vi "Get_WebService_Data.vi"(8 "error in (no error)":errorcluster, 11 "Class in":refnum<class "AB_WebService.lvclass">) -> (0 "error out":errorcluster, 2 "data":T1, 3 "class out":refnum<class "AB_WebService.lvclass">)   [LabVIEW 2020, in "AB_WebService.lvclass"]
uses:
  <vilib>/AppBuilder/AB_Classes/WebService/AB_WebService.lvclass
  <vilib>/AppBuilder/AB_Classes/WebService/AB_WebService.ctl
  <vilib>/AppBuilder/AB_Classes/WebService/AB_WebService.lvclass/AB_WebService.ctl
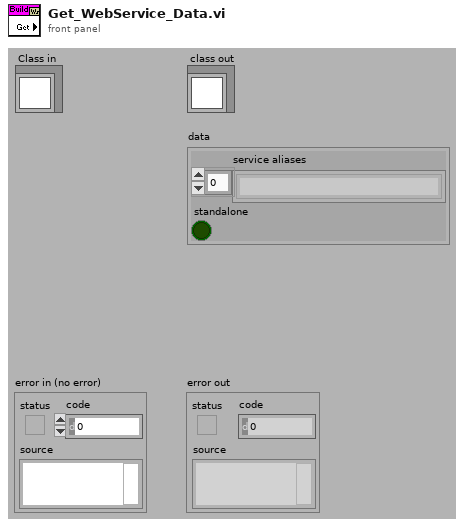
[diagram p1: front panel]
types:
  T1 = typedef "AB_WebService.ctl" = cluster{"service aliases":string[], "standalone":bool}
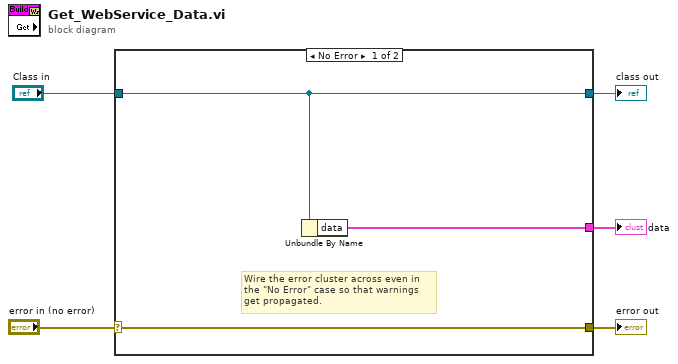
[diagram p0: block diagram]
diagram:
  n1 = case shown="No Error" "error in (no error)" {
    selector: "error in (no error)" -> [w8 w10]
    tunnel: [w8 w10] -> w4
    tunnel: [w6 _] -> w3
    tunnel: "Class in" -> [w7 w9]
    tunnel: [w7 w9] -> w1
    frame No Error {
      # "Wire the error cluster across even in the \"No Error\" case so that warnings get propagated."
      n2 = Unbundle By Name(w7) -> ("data"=w6:T1)
    }
    frame Error {
    }
  }
  "error out" <- w4
  "class out" <- w1
  "data" <- w3
